vi "SubVI_DriveForward_Auto.vi"(7 "PIDF":dbl[](array[numeric]), 9 "Inches to target":dbl=18.85 format="%#_13g", 10 "Speed":dbl=2000.0) -> ()   [LabVIEW 2017]
uses:
  <vilib>/Rock Robotics/WPI/ThirdParty/Phoenix-LabVIEW/Motor Controller/Controls/CTRE_Phoenix_MotorControl_FeedbackDevice.ctl
  <vilib>/Rock Robotics/WPI/ThirdParty/Phoenix-LabVIEW/Motor Controller/Controls/CTRE_Phoenix_MotorControl_ControlMode.ctl
  <vilib>/Rock Robotics/WPI/ThirdParty/Phoenix-LabVIEW/Motor Controller/Get/CTRE_Phoenix_MotorController_GetSelectedSensorData.vi
panel:
  in  "False = Encoders average True = Encoders reading seperately":bool
  out "Encoder Average":dbl
  out "Position(Right encoder)":dbl
  out "Position(Left encoder)":dbl
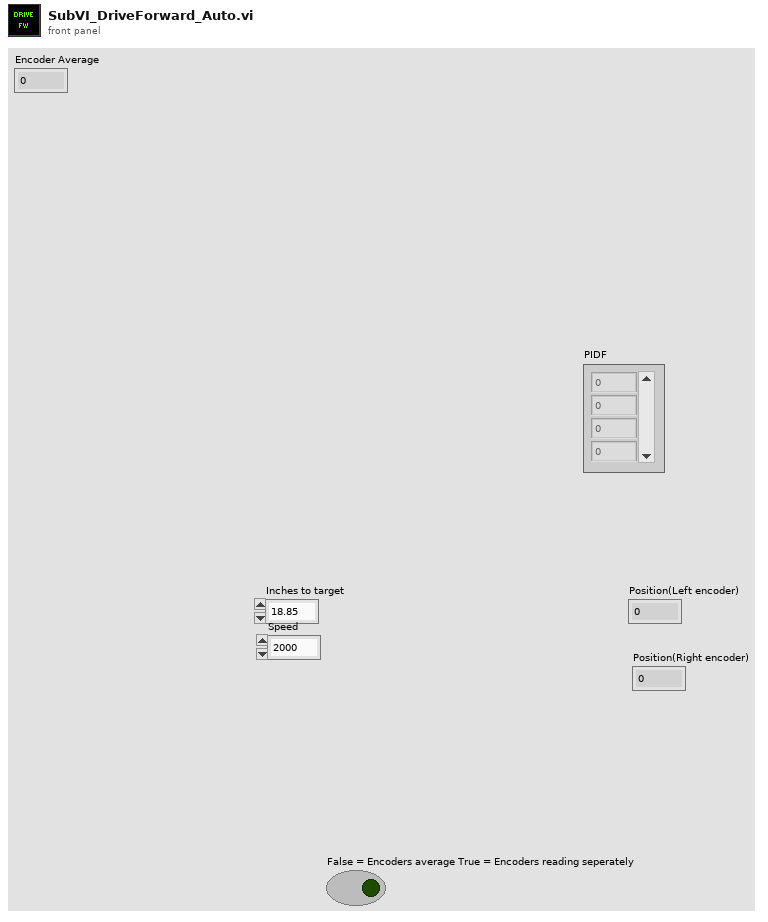
[diagram p1: front panel]
types:
  T1 = typedef "CTRE_Phoenix_MotorControl_FeedbackDevice.ctl" = i8
  T2 = typedef "WPI_MotorControlDeviceRef.ctl" = cluster{"DeviceStatus":errorcluster, "Type":T3, "PWM":cluster{"PWM Channel":T4, "DeadBand":T5}, "CAN":cluster{"Device Number":u8, "SetOutput VI Ref":variant, "GetOutput VI Ref":variant, "Enable VI Ref":variant, "Disable VI Ref":variant, "Data":variant}, "Invert":bool, "DIO PWM":cluster{"PWM \"Enable\" Channel":T4, "DIOChannel":T6, "PWM Rate":dbl}}
  T3 = typedef "WPI_MotorControlType.ctl" = enum16{"PWM", "CAN", "DIO PWM"}
  T4 = typedef "FPGA_DIOPWMChannel.ctl" = enum8{"PWM 0", "PWM 1", "PWM 2", "PWM 3", "PWM 4", "PWM 5", "PWM 6", "PWM 7", "PWM 8", "PWM 9", "PWM MXP 0", "PWM MXP 1", "PWM MXP 2", "PWM MXP 3", "PWM MXP 4", "PWM MXP 5", "PWM MXP 6", "PWM MXP 7", "PWM MXP 8", "PWM MXP 9", "Invalid"}
  T5 = typedef "WPI_PWMDeadband.ctl" = cluster{"Name":string, "maxPositivePwm":i32, "minPositivePwm":i32, "centerPwm":i32, "maxNegativePwm":i32, "minNegativePwm":i32, "angularRange":u16}
  T6 = typedef "FPGA_DIOChannel.ctl" = enum8{"DIO 0", "DIO 1", "DIO 2", "DIO 3", "DIO 4", "DIO 5", "DIO 6", "DIO 7", "DIO 8", "DIO 9", "DIO MXP 0", "DIO MXP 1", "DIO MXP 2", "DIO MXP 3", "DIO MXP 4", "DIO MXP 5", "DIO MXP 6", "DIO MXP 7", "DIO MXP 8", "DIO MXP 9", "DIO MXP 10", "DIO MXP 11", "DIO MXP 12", "DIO MXP 13", "DIO MXP 14", "DIO MXP 15", "SPI Port CS1", "SPI Port CS2", "SPI Port CS3", "SPI Port MISO", "SPI Port MOSI", "Invalid"}
  T7 = typedef "CTRE_Phoenix_MotorControl_ControlMode.ctl" = u16
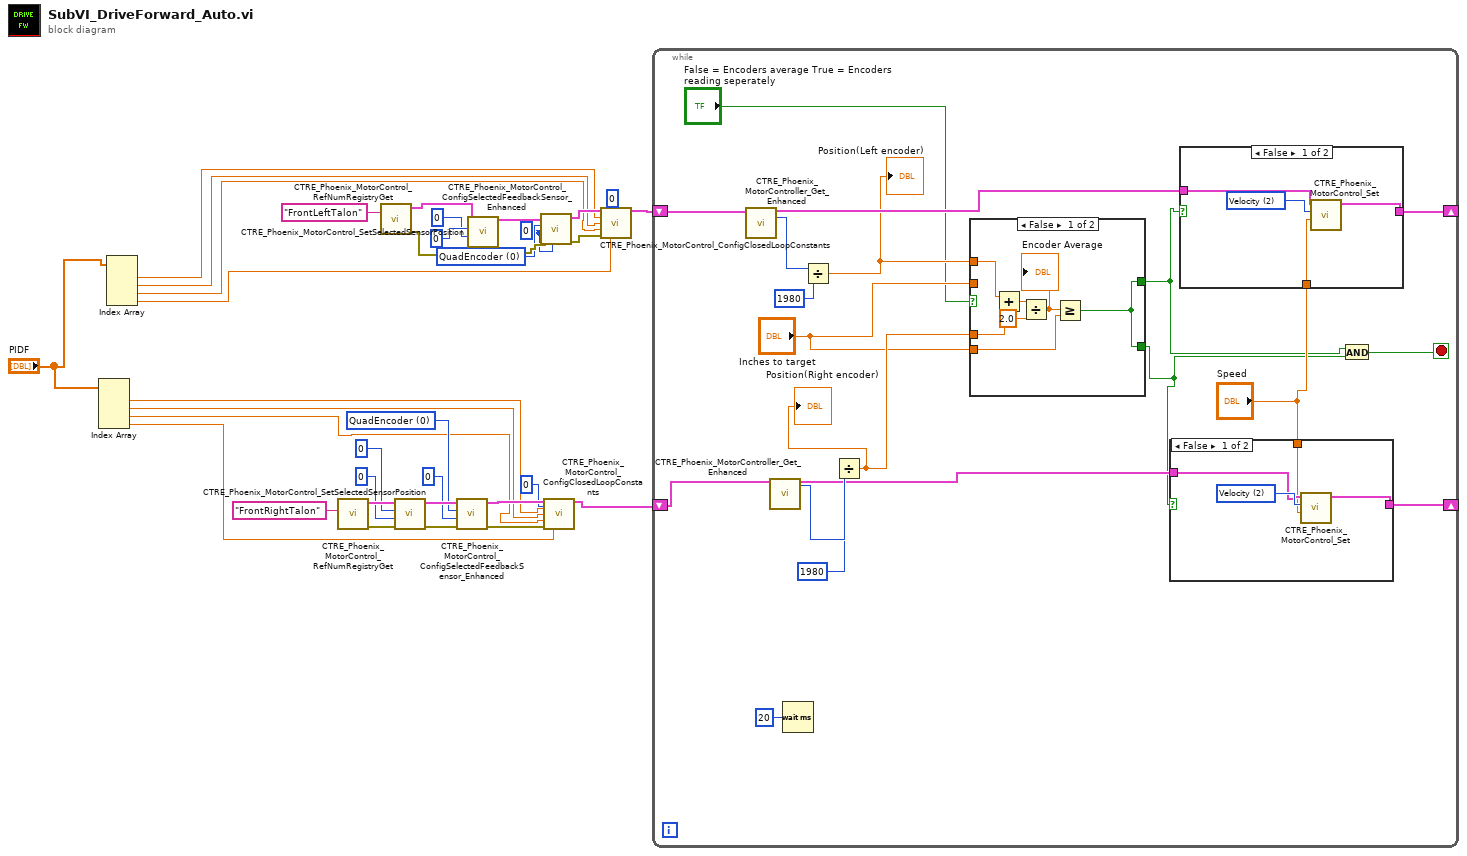
[diagram p0: block diagram]
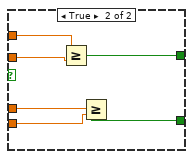
[diagram p2: hidden frame]
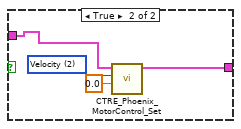
[diagram p3: hidden frame]
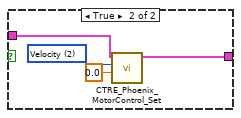
[diagram p4: hidden frame]
diagram:
  w14 = T1 0 items=["None"=-1, "QuadEncoder"=0, "Analog"=2, "Tachometer"=4, "Pulse Width Encoded Position"=8, "Sensor Sum (S0 + S1)"=9, "Sensor Difference (D0 - D1)"=10, "Remote Source 0"=11, "Remote Source 1"=12, "Software Emulated"=15] ("Feedback Device")
  w10 = 0 ("pidLoopIdx")
  w26 = T1 0 items=["None"=-1, "QuadEncoder"=0, "Analog"=2, "Tachometer"=4, "Pulse Width Encoded Position"=8, "Sensor Sum (S0 + S1)"=9, "Sensor Difference (D0 - D1)"=10, "Remote Source 0"=11, "Remote Source 1"=12, "Software Emulated"=15] ("Feedback Device")
  n1 = Index Array(array="PIDF") -> (element #1=w4:dbl, element #2=w3:dbl, element #3=w2:dbl, element #4=w1:dbl)  [unwired: 4 in]
  n2 = Index Array(array="PIDF") -> (element #1=w8:dbl, element #2=w7:dbl, element #3=w6:dbl, element #4=w5:dbl)  [unwired: 4 in]
  n3 = call <vilib>:"CTRE_Phoenix_MotorControl_RefNumRegistryGet.vi"("refnum name"="FrontRightTalon") -> ("error out"=w21:errorcluster, "PhoenixMotorControlDevRef"=w22:T2)  [unwired: 9 in]
  n4 = call <vilib>:"CTRE_Phoenix_MotorControl_RefNumRegistryGet.vi"("refnum name"="FrontLeftTalon") -> ("error out"=w33:errorcluster, "PhoenixMotorControlDevRef"=w34:T2)  [unwired: 9 in]
  n5 = call <vilib>:"CTRE_Phoenix_MotorControl_SetSelectedSensorPosition.vi"("error in (no error)"=w21, "pidLoopIdx"=u32 0, "New Sensor Position"=0, "PhoenixMotorControlDevRef"=w22) -> ("error out"=w16:errorcluster, "PhoenixMotorControlDevRef"=w18:T2)  [unwired: 6 in]
  n6 = call <vilib>:"CTRE_Phoenix_MotorControl_ConfigSelectedFeedbackSensor_Enhanced.vi"("error in (no error)"=w16, "pidLoopIdx"=0, "Feedback Device"=w14, "PhoenixMotorControlDevRef"=w18) -> ("error out"=w15:errorcluster, "PhoenixMotorControlDevRef"=w17:T2)  [unwired: 6 in]
  n7 = call <vilib>:"CTRE_Phoenix_MotorControl_SetSelectedSensorPosition.vi"("error in (no error)"=w33, "pidLoopIdx"=u32 0, "New Sensor Position"=0, "PhoenixMotorControlDevRef"=w34) -> ("error out"=w28:errorcluster, "PhoenixMotorControlDevRef"=w30:T2)  [unwired: 6 in]
  n8 = call <vilib>:"CTRE_Phoenix_MotorControl_ConfigSelectedFeedbackSensor_Enhanced.vi"("timeoutMs"=w10, "error in (no error)"=w28, "pidLoopIdx"=w10, "Feedback Device"=w26, "PhoenixMotorControlDevRef"=w30) -> ("error out"=w27:errorcluster, "PhoenixMotorControlDevRef"=w29:T2)  [unwired: 5 in]
  n9 = call <vilib>:"CTRE_Phoenix_MotorControl_ConfigClosedLoopConstants.vi"("PhoenixMotorControlDevRef"=w17, "slotIdx"=0, "P"=w4, "I"=w3, "D"=w2, "error in (no error)"=w15, "F"=w1) -> ("PhoenixMotorControlDevRef"=w11:T2)  [unwired: 7 in, 1 out]
  n10 = call <vilib>:"CTRE_Phoenix_MotorControl_ConfigClosedLoopConstants.vi"("PhoenixMotorControlDevRef"=w29, "slotIdx"=0, "P"=w8, "I"=w7, "D"=w6, "error in (no error)"=w27, "F"=w5) -> ("PhoenixMotorControlDevRef"=w25:T2)  [unwired: 7 in, 1 out]
  n11 = while {
    shift-right: [w51] -> _
    shift-left: w25 -> [w50]
    shift-right: [w48] -> _
    shift-left: w11 -> [w45]
    stop <- w42 stop-if-true
    n12 = call-poly <vilib>:"CTRE_Phoenix_MotorController_Get_Enhanced.vi"("PhoenixMotorControlDevRef"=w50) -> ("PhoenixMotorControlDevRef"=w52:T2, "Position (Raw Sensor Units)"=w54:i32)  [unwired: 11 in, 2 out]
    n13 = call-poly <vilib>:"CTRE_Phoenix_MotorController_Get_Enhanced.vi"("PhoenixMotorControlDevRef"=w45) -> ("PhoenixMotorControlDevRef"=w44:T2, "Position (Raw Sensor Units)"=w46:i32)  [unwired: 11 in, 2 out]
    n14 = Wait (ms)(milliseconds to wait=u32 20) -> ()  [unwired: 1 out]
    n15 = Divide(x=w54, y=1980) -> (x/y=w41:dbl)
    "Position(Left encoder)" <- w41
    n16 = Divide(x=w46, y=1980) -> (x/y=w40:dbl)
    "Position(Right encoder)" <- w40
    n17 = case shown="False" "False = Encoders average True = Encoders reading seperately" {
      tunnel: w41 -> [w61 w63]
      tunnel: "Inches to target" -> [w55 w65]
      tunnel: w40 -> [w56 w64]
      tunnel: [w58 w67] -> w38
      tunnel: [w58 w66] -> w37
      tunnel: "Inches to target" -> [_ w62]
      frame False {
        n18 = Add(x=w61, y=w56) -> (x+y=w60:dbl)
        n19 = Divide(x=w60, y=2.0) -> (x/y=w59:dbl)
        "Encoder Average" <- w59
        n20 = Greater Or Equal?(x=w59, y=w55) -> (x >= y?=w58:bool)
      }
      frame True {
        n21 = Greater Or Equal?(x=w63, y=w62) -> (x >= y?=w67:bool)
        n22 = Greater Or Equal?(x=w64, y=w65) -> (x >= y?=w66:bool)
      }
    }
    n23 = case shown="False" w37 {
      tunnel: [w70 w73] -> w48
      tunnel: w44 -> [w69 w72]
      tunnel: "Speed" -> [w68 _]
      frame False {
        w71 = T7 2 items=["PercentOutput"=0, "Position"=1, "Velocity"=2, "Current"=3, "Follower"=5, "MotionProfile"=6, "MotionMagic"=7, "MotionMagicArc"=8, "MotionProfileArc"=10, "Disabled"=15] ("Control Mode")
        n24 = call <vilib>:"CTRE_Phoenix_MotorControl_Set.vi"("Output"=w68, "Control Mode"=w71, "PhoenixMotorControlDevRef"=w69) -> ("PhoenixMotorControlDevRef"=w70:T2)  [unwired: 7 in, 1 out]
      }
      frame True {
        w74 = T7 2 items=["PercentOutput"=0, "Position"=1, "Velocity"=2, "Current"=3, "Follower"=5, "MotionProfile"=6, "MotionMagic"=7, "MotionMagicArc"=8, "MotionProfileArc"=10, "Disabled"=15] ("Control Mode")
        n25 = call <vilib>:"CTRE_Phoenix_MotorControl_Set.vi"("Output"=0.0, "Control Mode"=w74, "PhoenixMotorControlDevRef"=w72) -> ("PhoenixMotorControlDevRef"=w73:T2)  [unwired: 7 in, 1 out]
      }
    }
    n26 = case shown="False" w38 {
      tunnel: w52 -> [w78 w83]
      tunnel: [w77 w80] -> w51
      tunnel: "Speed" -> [w76 _]
      frame False {
        w79 = T7 2 items=["PercentOutput"=0, "Position"=1, "Velocity"=2, "Current"=3, "Follower"=5, "MotionProfile"=6, "MotionMagic"=7, "MotionMagicArc"=8, "MotionProfileArc"=10, "Disabled"=15] ("Control Mode")
        n27 = call <vilib>:"CTRE_Phoenix_MotorControl_Set.vi"("Output"=w76, "Control Mode"=w79, "PhoenixMotorControlDevRef"=w78) -> ("PhoenixMotorControlDevRef"=w77:T2)  [unwired: 7 in, 1 out]
      }
      frame True {
        w81 = T7 2 items=["PercentOutput"=0, "Position"=1, "Velocity"=2, "Current"=3, "Follower"=5, "MotionProfile"=6, "MotionMagic"=7, "MotionMagicArc"=8, "MotionProfileArc"=10, "Disabled"=15] ("Control Mode")
        n28 = call <vilib>:"CTRE_Phoenix_MotorControl_Set.vi"("Output"=0.0, "Control Mode"=w81, "PhoenixMotorControlDevRef"=w83) -> ("PhoenixMotorControlDevRef"=w80:T2)  [unwired: 7 in, 1 out]
      }
    }
    n29 = And(x=w38, y=w37) -> (x .and. y?=w42:bool)
  }
